vi "UI - Read IO Variables.vi"(8 "error in (no error)":errorcluster, 11 "IO References":T1) -> (0 "error out":errorcluster, 2 "Control Output Values":dbl[](array[numeric]), 3 "Control Input Values":dbl[](array[numeric]))   [LabVIEW 2014]
uses:
  Controls/IO References.ctl
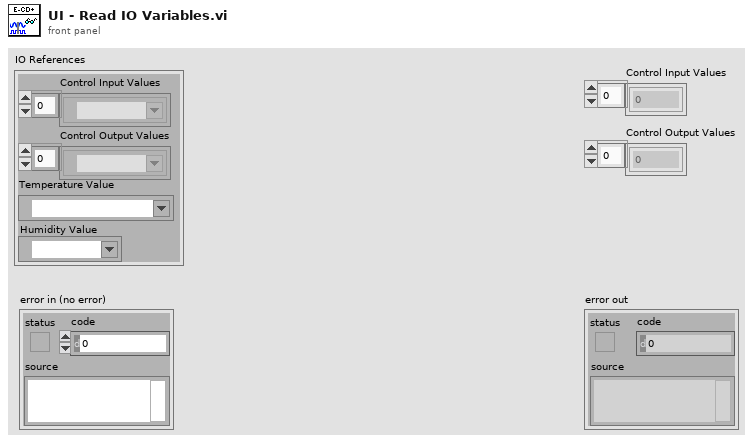
[diagram p1: front panel]
types:
  T1 = typedef "IO References.ctl" = cluster{"Control Input Values":refnum<k21>[], "Control Output Values":refnum<k21>[], "Temperature Value":refnum<k21>, "Humidity Value":refnum<k21>}
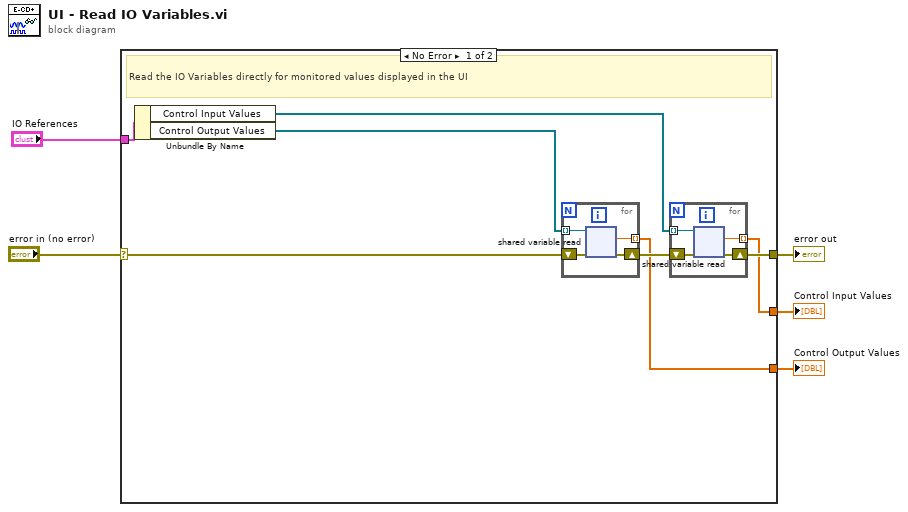
[diagram p0: block diagram]
diagram:
  n1 = case shown="No Error" "error in (no error)" {
    selector: "error in (no error)" -> [w6 w22]
    tunnel: "IO References" -> [w13 _]
    tunnel: [w9 w22] -> w4
    tunnel: [w8 _] -> w3
    tunnel: [w7 _] -> w2
    frame No Error {
      # "Read the IO Variables directly for monitored values displayed in the UI"
      n2 = Unbundle By Name(w13) -> ("Control Input Values"=w10:refnum<k21>[], "Control Output Values"=w12:refnum<k21>[])
      n3 = for {
        shift-right: [w19] -> w11
        shift-left: w6 -> [w20]
        tunnel: w12 -> [w21] mode=indexing
        tunnel: [w18] -> w8 mode=indexing
        n4 = shared-variable-read(w21, w20) -> (w19:errorcluster, w18:dbl)  [unwired: 2 out]
      }
      n5 = for {
        shift-right: [w15] -> w9
        shift-left: w11 -> [w16]
        tunnel: w10 -> [w17] mode=indexing
        tunnel: [w14] -> w7 mode=indexing
        n6 = shared-variable-read(w17, w16) -> (w15:errorcluster, w14:dbl)  [unwired: 2 out]
      }
    }
    frame Error {
      # "Error"
    }
  }
  "error out" <- w4
  "Control Input Values" <- w2
  "Control Output Values" <- w3
